vi "TestFlux.vi"(8 "error in (no error)":errorcluster, 11 "reference in":refnum<class "Flux_Capacitor.lvclass">) -> (0 "error out":errorcluster, 1 "OK":bool, 3 "reference in":refnum<class "Flux_Capacitor.lvclass">)   [LabVIEW 2022 SP3, in "Flux_Capacitor.lvlib" / "Flux_Capacitor.lvclass"]
uses:
  Flux_Capacitor.lvclass
  Components/ViPER.lvlibp/ViPER.lvclass
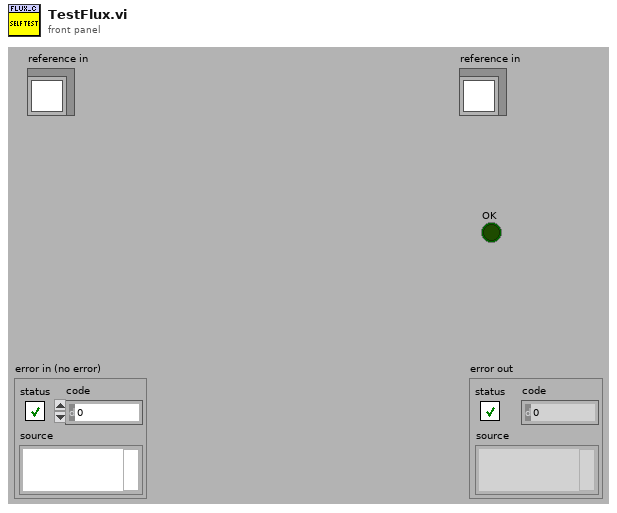
[diagram p1: front panel]
types:
  T1 = typedef "Flux_Capacitor.lvlib/Flux_Capacitor.lvclass/ObjectAttributes.ctl" = cluster{"Config":T2, "T Sensors":T3[], "Temp_DegC":dbl[], "Temp_Raw":u64[], "RTC":timestamp, "Flux":bool, "Time":timestamp, "RTC_Live":timestamp}
  T2 = typedef "Flux_Capacitor.lvlib/Flux_Capacitor.lvclass/Config.ctl" = cluster{"default":string}
  T3 = typedef "Flux_Capacitor.lvlib/Flux_Capacitor.lvclass/TempSensor.ctl" = enum16{"1", "2", "3"}
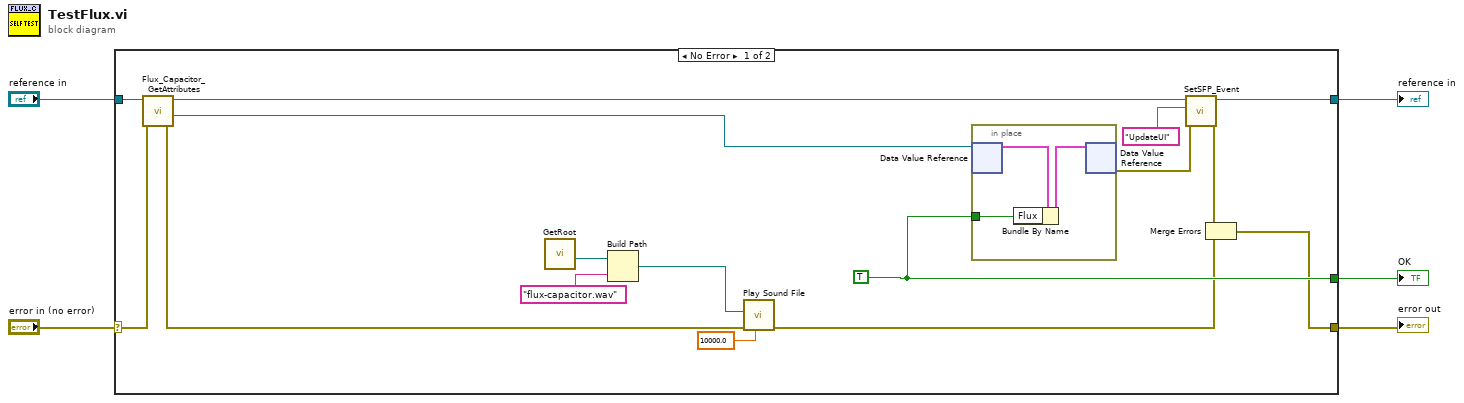
[diagram p0: block diagram]
diagram:
  n1 = case shown="No Error" "error in (no error)" {
    selector: "error in (no error)" -> [w21 w26]
    tunnel: [w7 w26] -> w4
    tunnel: [w6 w25] -> w2
    tunnel: "reference in" -> [w20 w25]
    tunnel: [w15 _] -> w1
    frame No Error {
      w15 = TRUE
      n2 = call "Flux_Capacitor_GetAttributes.vi"("error in (no error)"=w21, "reference in"=w20) -> ("error out"=w9:errorcluster, "DataRef"=w16:refnum<data-value>, "reference out"=w8:refnum<class "Flux_Capacitor.lvclass">)  [unwired: 6 in, 1 out]
      n3 = call "GetRoot.vi"() -> ("Root"=w13:path)  [unwired: 10 in, 1 out]
      n4 = Build Path(base path=w13, name or relative path="flux-capacitor.wav") -> (appended path=w11:path)
      n5 = call <vilib>:"Play Sound File.vi"("timeout (sec)"=10000.0, "error in (no error)"=w9, "path"=w11) -> ("error out"=w10:errorcluster)  [unwired: 7 in, 1 out]
      n6 = in-place {
        in-place-border: w15 -> [w22]
        n7 = in-place-dvr #1(w16) -> (w24:T1)  [unwired: 1 out]
        n8 = Bundle By Name(cluster=w24, "Flux"=w22) -> (w23:T1)
        n9 = in-place-dvr #1(w23) -> (w19:errorcluster)  [unwired: 1 out]
      }
      n10 = call-dynamic "SetSFP_Event.vi"("error in (no error)"=w19, "msg"="UpdateUI", "reference in"=w8) -> ("error out"=w18:errorcluster, "reference out"=w6:refnum<class "Flux_Capacitor.lvclass">)  [unwired: 7 in]
      n11 = Merge Errors(w18, w10) -> (w7:errorcluster)
    }
    frame Error {
    }
  }
  "error out" <- w4
  "reference in" <- w2
  "OK" <- w1
